vi "Item_OnCommand.vi"(10 "Command ID":string, 11 "Object":T1) -> ()   [LabVIEW 2020, in "Message Rescripter.lvlib"]
uses:
  Message Rescripter.lvlib
  MessageMakerProvider/_Message Maker/Message Maker.lvlib
  Classes/Coupled Message Rescripter/Coupled Message Rescripter.lvclass
  MessageMakerProvider/_Message Maker/_Maker Classes/Target Method Prototyper/Target Method Prototyper.lvclass
  MessageMakerProvider/_Message Maker/_Maker Classes/Message Scripter/Message Scripter.lvclass
  Classes/Abstract Message Rescripter/Abstract Message Rescripter.lvclass
  MessageMakerProvider/_Message Maker/_Maker Classes/User Defined Prototype/User Defined Prototype.lvclass
  MessageMakerProvider/_Message Maker/_Maker Classes/Reference Method Prototyper/Reference Method Prototyper.lvclass
  Classes/Concrete Message Rescripter/Concrete Message Rescripter.lvclass
  MessageMakerProvider/_Message Maker/_Maker Classes/Target Method Icon Reader/Target Method Icon Reader.lvclass
  MessageMakerProvider/AFPP Shared/AFPP Shared.lvlib
  <vilib>/ErrorRing/Error Ring.xnode
  MessageMakerProvider/AFPP Shared/Validation Mode.ctl
  <vilib>/Utility/error.llb/Error Cluster From Error Code.vi
  MessageMakerProvider/_Message Maker/_Maker Classes/Abstract Icon Prototyper/Abstract Icon Prototyper.lvclass
  <resource>/Framework/Providers/API/ItemRef.ctl
panel:
  out "error out":errorcluster
  in  "error in":errorcluster
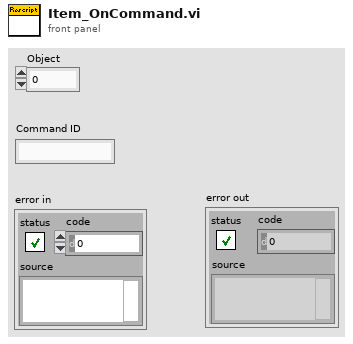
[diagram p1: front panel]
types:
  T1 = typedef "ItemRef.ctl" = u64
  T2 = typedef "AFPP Shared.lvlib/Validation Mode.ctl" = enum16{"An Actor Library", "A Target Tag"}
  T3 = enum16{"Invalid", "Abstract", "Concrete", "Standard"}
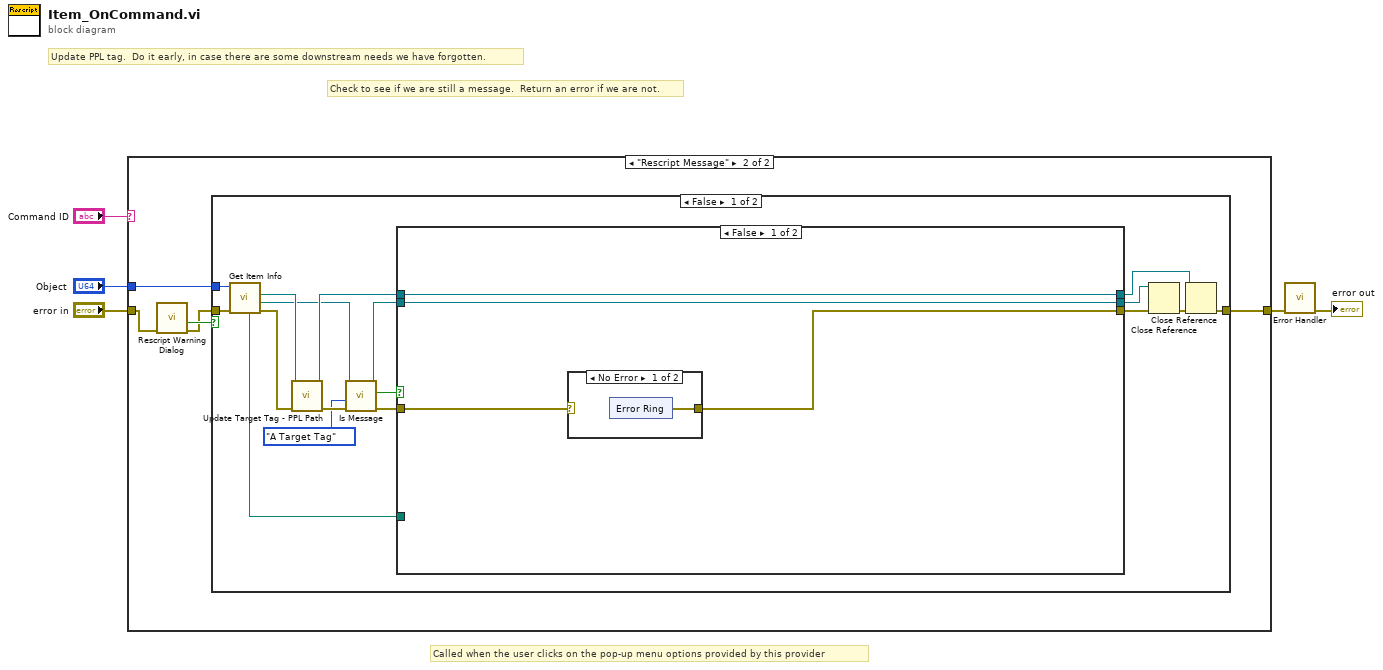
[diagram p0: block diagram]
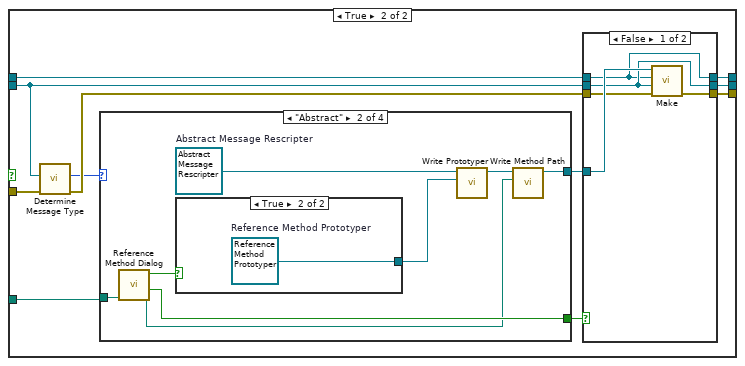
[diagram p4: hidden frame]
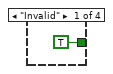
[diagram p6: hidden frame]
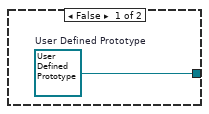
[diagram p7: hidden frame]
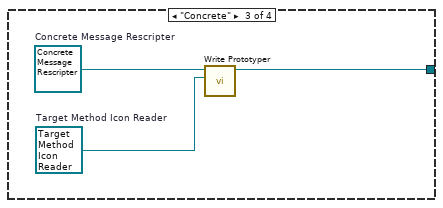
[diagram p8: hidden frame]
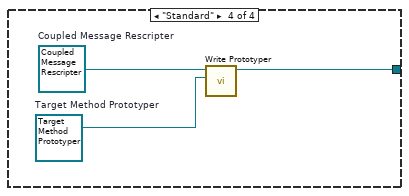
[diagram p9: hidden frame]
diagram:
  # "Check to see if we are still a message.  Return an error if we are not."
  # "Update PPL tag.  Do it early, in case there are some downstream needs we have forgotten."
  # "Called when the user clicks on the pop-up menu options provided by this provider"
  n1 = case shown="\"Rescript Message\"" "Command ID" {
    tunnel: "error in" -> [w6 w8]
    tunnel: [w6 w10] -> w2
    tunnel: "Object" -> [_ w11]
    frame Default {
    }
    frame "Rescript Message" {
      n2 = call "Rescript Warning Dialog.vi"("error in (no error)"=w8) -> ("error out"=w7:errorcluster, "Cancelled?"=w9:bool)  [unwired: 9 in]
      n3 = case shown="False" w9 {
        tunnel: w11 -> [w28 _]
        tunnel: w7 -> [w27 w76]
        tunnel: [w15 w76] -> w10
        frame False {
          n4 = call "Get Item Info.vi"("error in (no error)"=w27, "Object"=w28) -> ("error out"=w24:errorcluster, "Item Refnum"=w20:refnum<vi>, "Target"=w23:refnum<vi>, "Project Path"=w25:path)  [unwired: 5 in, 1 out]
          n5 = call "Update Target Tag - PPL Path.vi"("error in (no error)"=w24, "Target"=w23) -> ("error out"=w21:errorcluster, "dup Target"=w22:refnum<vi>)  [unwired: 7 in, 1 out]
          n6 = call "Is Message.vi"("error in (no error)"=w21, "Validation"=Validation_Mode."A Target Tag", "ProjectItem in"=w20) -> ("error out"=w18:errorcluster, "Is Message"=w17:bool, "ProjectItem out"=w19:refnum<vi>)  [unwired: 6 in]
          n7 = case shown="False" w17 {
            tunnel: [w29 w50] -> w26
            tunnel: w25 -> [_ w46]
            tunnel: w22 -> [w32 w44]
            tunnel: w19 -> [w31 w43]
            tunnel: w18 -> [w30 w42]
            tunnel: [w31 w41] -> w14
            tunnel: [w32 w40] -> w13
            frame False {
              n8 = case shown="No Error" w30 {
                selector: w30 -> [_ w39]
                tunnel: [w33 w39] -> w29
                frame No Error {
                  n9 = xnode "Error Ring"() -> ("error out"=w33:errorcluster)
                }
                frame Error {
                }
              }
            }
            frame True {
              n10 = call "Determine Message Type.vi"("error in"=w42, "Item Refnum"=w43) -> ("error out"=w48:errorcluster, "Enum"=w47:T3)  [unwired: 8 in]
              n11 = case shown="\"Abstract\"" w47 {
                tunnel: [_ w61 w72 w73] -> w49
                tunnel: w46 -> [_ w65 _ _]
                tunnel: [TRUE ("Cancelled?") w63 _ _] -> w45
                frame "Invalid" {
                }
                frame "Abstract" {
                  w67 = refnum<class "Abstract Message Rescripter.lvclass"> refnum  # Abstract Message Rescripter
                  n12 = call "Reference Method Dialog.vi"("Start Path"=w65) -> ("Path out"=w60:path, "Cancelled?"=w63:bool, "Use Reference Method out"=w66:bool)  [unwired: 8 in]
                  n13 = case shown="True" w66 {
                    tunnel: [w68 w69] -> w64
                    frame False {
                      w68 = refnum<class "User Defined Prototype.lvclass"> refnum  # User Defined Prototype
                    }
                    frame True {
                      w69 = refnum<class "Reference Method Prototyper.lvclass"> refnum  # Reference Method Prototyper
                    }
                  }
                  n14 = call "Write Prototyper.vi"("Prototyper"=w64, "Message Scripter in"=w67) -> ("Message Scripter out"=w62:refnum<class "Abstract Message Rescripter.lvclass">)  [unwired: 9 in]
                  n15 = call "Write Method Path.vi"("Method Path"=w60, "Message Scripter in"=w62) -> ("Message Scripter out"=w61:refnum<class "Abstract Message Rescripter.lvclass">)  [unwired: 9 in]
                }
                frame "Concrete" {
                  w70 = refnum<class "Target Method Icon Reader.lvclass"> refnum  # Target Method Icon Reader
                  w71 = refnum<class "Concrete Message Rescripter.lvclass"> refnum  # Concrete Message Rescripter
                  n16 = call "Write Prototyper.vi"("Prototyper"=w70, "Message Scripter in"=w71) -> ("Message Scripter out"=w72:refnum<class "Concrete Message Rescripter.lvclass">)  [unwired: 9 in]
                }
                frame "Standard" {
                  w75 = refnum<class "Target Method Prototyper.lvclass"> refnum  # Target Method Prototyper
                  w74 = refnum<class "Coupled Message Rescripter.lvclass"> refnum  # Coupled Message Rescripter
                  n17 = call "Write Prototyper.vi"("Prototyper"=w75, "Message Scripter in"=w74) -> ("Message Scripter out"=w73:refnum<class "Coupled Message Rescripter.lvclass">)  [unwired: 9 in]
                }
              }
              n18 = case shown="False" w45 {
                tunnel: w44 -> [w51 w56]
                tunnel: [w55 w58] -> w50
                tunnel: w49 -> [w54 _]
                tunnel: w43 -> [w52 w57]
                tunnel: w48 -> [w53 w58]
                tunnel: [w52 w57] -> w41
                tunnel: [w51 w56] -> w40
                frame False {
                  n19 = call-dynamic "Make.vi"("error in (no error)"=w53, "Item Refnum"=w52, "Target"=w51, "Message Scripter"=w54) -> ("error out"=w55:errorcluster)  [unwired: 6 in, 1 out]
                }
                frame True {
                }
              }
            }
          }
          n20 = Close Reference(reference=w14, error in (no error)=w26) -> (error out=w16:errorcluster)
          n21 = Close Reference(reference=w13, error in (no error)=w16) -> (error out=w15:errorcluster)
        }
        frame True {
        }
      }
    }
  }
  n22 = call "Error Handler.vi"("error in (no error)"=w2) -> ("error out"=→"error out":errorcluster)  [unwired: 10 in]
